vi "Autosetup.vi"(8 "error in (no error)":errorcluster, 11 "EDU-X-1002A in":refnum<class "EDU-X-1002A.lvclass">) -> (0 "error out":errorcluster, 3 "EDU-X-1002A out":refnum<class "EDU-X-1002A.lvclass">)   [LabVIEW 2020, in "Controlador.lvlib" / "EDU-X-1002A.lvclass"]
uses:
  EDU-X-1002A.lvclass
  C:/Users/scrap/Fork/Modulo_Cloneable_DQMH/Libraries/Controlador/Class/Osciloscope/Osciloscope.lvclass
  Osciloscope/Osciloscope.lvclass/Osciloscope.ctl
  Osciloscope/Read COM.vi
  <instrlib>/Agilent 2000 3000 X-Series/Agilent 2000 3000 X-Series.lvlib
  Osciloscope/Osciloscope.lvclass
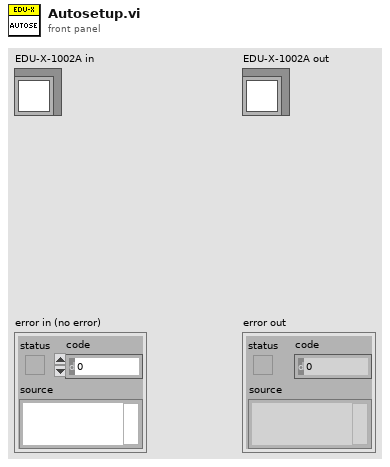
[diagram p1: front panel]
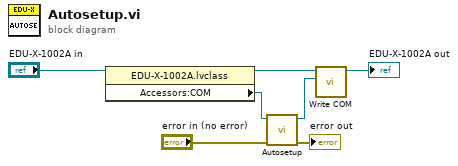
[diagram p0: block diagram]
diagram:
  n1 = property class="EDU-X-1002A.lvclass"(reference="EDU-X-1002A in") -> (reference out=w7:refnum<class "EDU-X-1002A.lvclass">, "Accessors:COM"=w6:refnum<visa-resource-name>)  [unwired: 1 in, 1 out]
  n2 = call <instrlib>:"Autosetup.vi"("error in (no error)"="error in (no error)", "VISA resource name"=w6) -> ("error out"=→"error out":errorcluster, "VISA resource name out"=w3:refnum<visa-resource-name>)  [unwired: 8 in]
  n3 = call "Write COM.vi"("COM"=w3, "Osciloscope in"=w7) -> ("Osciloscope out"=→"EDU-X-1002A out":refnum<class "EDU-X-1002A.lvclass">)  [unwired: 8 in, 1 out]
